vi "READ NEO values.vi"(8 "error in (no error)":errorcluster, 10 "RefName":string, 11 "MotorControlDevRef":T1) -> (0 "error out":errorcluster, 3 "MotorControlDevRef out":T1)   [LabVIEW 2020]
uses:
  <vilib>/Rock Robotics/WPI/MotorControl/WPI_MotorControlDeviceRef.ctl
  <vilib>/Rock Robotics/WPI/MotorControl/WPI_MotorControlType.ctl
  <vilib>/Rock Robotics/SystemInterfaces/DIO/FPGA_DIOPWMChannel.ctl
  <vilib>/Rock Robotics/WPI/PWM/WPI_PWMDeadband.ctl
  <vilib>/Rock Robotics/SystemInterfaces/DIO/FPGA_DIOChannel.ctl
  <vilib>/Rock Robotics/Network Tables/NT Write Number.vi
  <vilib>/Rock Robotics/Network Tables/NT Write Boolean.vi
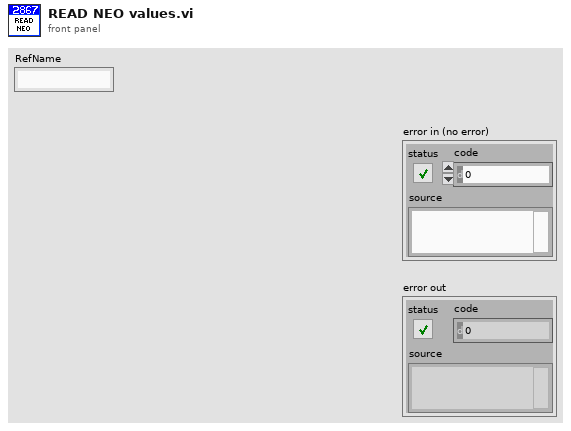
[diagram p1: front panel]
types:
  T1 = typedef "WPI_MotorControlDeviceRef.ctl" = cluster{"DeviceStatus":errorcluster, "Type":T2, "PWM":cluster{"PWM Channel":T3, "DeadBand":T4}, "CAN":cluster{"Device Number":u8, "SetOutput VI Ref":variant, "GetOutput VI Ref":variant, "Enable VI Ref":variant, "Disable VI Ref":variant, "Data":variant}, "Invert":bool, "DIO PWM":cluster{"PWM \"Enable\" Channel":T3, "DIOChannel":T5, "PWM Rate":dbl}}
  T2 = typedef "WPI_MotorControlType.ctl" = enum16{"PWM", "CAN", "DIO PWM"}
  T3 = typedef "FPGA_DIOPWMChannel.ctl" = enum8{"PWM 0", "PWM 1", "PWM 2", "PWM 3", "PWM 4", "PWM 5", "PWM 6", "PWM 7", "PWM 8", "PWM 9", "PWM MXP 0", "PWM MXP 1", "PWM MXP 2", "PWM MXP 3", "PWM MXP 4", "PWM MXP 5", "PWM MXP 6", "PWM MXP 7", "PWM MXP 8", "PWM MXP 9", "Invalid"}
  T4 = typedef "WPI_PWMDeadband.ctl" = cluster{"Name":string, "maxPositivePwm":i32, "minPositivePwm":i32, "centerPwm":i32, "maxNegativePwm":i32, "minNegativePwm":i32, "angularRange":u16}
  T5 = typedef "FPGA_DIOChannel.ctl" = enum8{"DIO 0", "DIO 1", "DIO 2", "DIO 3", "DIO 4", "DIO 5", "DIO 6", "DIO 7", "DIO 8", "DIO 9", "DIO MXP 0", "DIO MXP 1", "DIO MXP 2", "DIO MXP 3", "DIO MXP 4", "DIO MXP 5", "DIO MXP 6", "DIO MXP 7", "DIO MXP 8", "DIO MXP 9", "DIO MXP 10", "DIO MXP 11", "DIO MXP 12", "DIO MXP 13", "DIO MXP 14", "DIO MXP 15", "SPI Port CS1", "SPI Port CS2", "SPI Port CS3", "SPI Port MISO", "SPI Port MOSI", "Invalid"}
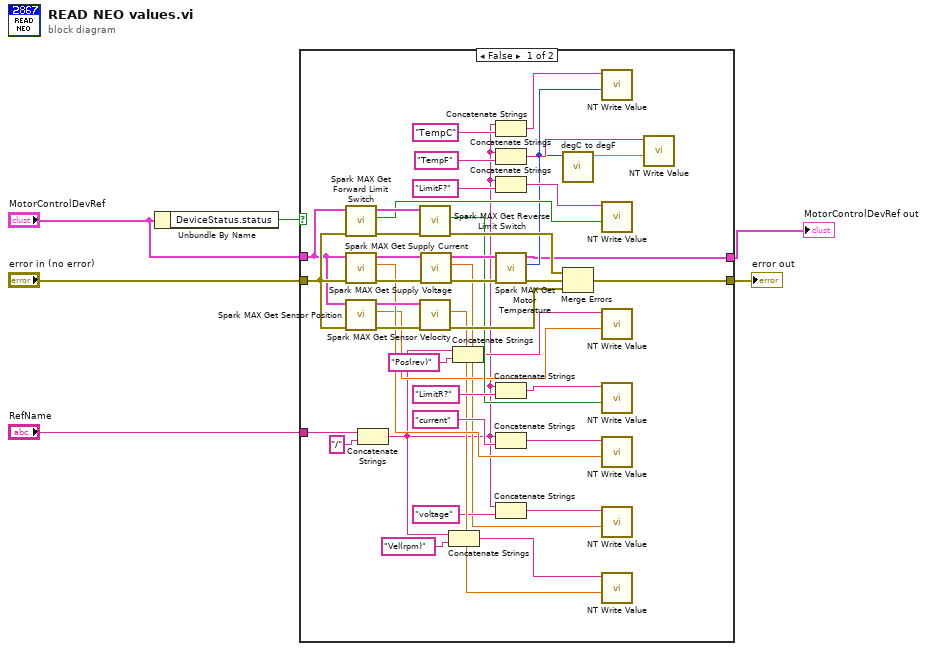
[diagram p0: block diagram]
diagram:
  n1 = Unbundle By Name("MotorControlDevRef") -> ("DeviceStatus.status"=w2:bool)
  n2 = case shown="False" w2 {
    tunnel: "RefName" -> [w48 _]
    tunnel: "error in (no error)" -> [w47 w49]
    tunnel: [w46 w49] -> w4
    tunnel: "MotorControlDevRef" -> [w45 w50]
    tunnel: [w7 w50] -> w1
    frame False {
      n3 = call <vilib>:"Spark MAX Get Forward Limit Switch.vi"("error in (no error)"=w47, "MotorControlDevRef in"=w45) -> ("error out"=w43:errorcluster, "Hard Limit Fwd"=w31:bool, "MotorControlDevRef out"=w40:T1)  [unwired: 6 in, 1 out]
      n4 = call <vilib>:"Spark MAX Get Supply Current.vi"("error in (no error)"=w47, "MotorControlDevRef in"=w45) -> ("error out"=w42:errorcluster, "Current"=w24:dbl, "MotorControlDevRef out"=w38:T1)  [unwired: 6 in, 1 out]
      n5 = call <vilib>:"Spark MAX Get Sensor Position.vi"("error in (no error)"=w47, "MotorControlDevRef in"=w45) -> ("error out"=w44:errorcluster, "Sensor Position"=w21:dbl, "MotorControlDevRef out"=w39:T1)  [unwired: 6 in, 1 out]
      n6 = Concatenate Strings(w48, "/" ("string")) -> (w8:string)
      n7 = call <vilib>:"Spark MAX Get Reverse Limit Switch.vi"("error in (no error)"=w43, "MotorControlDevRef in"=w40) -> ("error out"=w35:errorcluster, "Hard Limit Rev"=w27:bool)  [unwired: 6 in, 2 out]
      n8 = call <vilib>:"Spark MAX Get Sensor Velocity.vi"("error in (no error)"=w44, "MotorControlDevRef in"=w39) -> ("error out"=w36:errorcluster, "Sensor Velocity"=w18:dbl)  [unwired: 6 in, 2 out]
      n9 = call <vilib>:"Spark MAX Get Supply Voltage.vi"("error in (no error)"=w42, "MotorControlDevRef in"=w38) -> ("error out"=w41:errorcluster, "Voltage"=w15:dbl, "MotorControlDevRef out"=w37:T1)  [unwired: 6 in, 1 out]
      n10 = Concatenate Strings(w8, "Vel(rpm)" ("string")) -> (w20:string)
      n11 = Concatenate Strings(w8, "Pos(rev)" ("string")) -> (w23:string)
      n12 = Concatenate Strings(w8, "TempC" ("string")) -> (w14:string)
      n13 = Concatenate Strings(w8, "TempF" ("string")) -> (w12:string)
      n14 = Concatenate Strings(w8, "LimitF?" ("string")) -> (w32:string)
      n15 = call <vilib>:"Spark MAX Get Motor Temperature.vi"("error in (no error)"=w41, "MotorControlDevRef in"=w37) -> ("error out"=w34:errorcluster, "Motor Temperature"=w10:u8, "MotorControlDevRef out"=w7:T1)  [unwired: 6 in, 1 out]
      n16 = Concatenate Strings(w8, "LimitR?" ("string")) -> (w29:string)
      n17 = Concatenate Strings(w8, "current" ("string")) -> (w26:string)
      n18 = Concatenate Strings(w8, "voltage" ("string")) -> (w17:string)
      n19 = call "degC to degF.vi"("degreesC"=w10) -> ("degreesF"=w9:dbl)  [unwired: 10 in]
      n20 = Merge Errors(w35, w34, w36) -> (w46:errorcluster)
      n21 = call-poly <vilib>:"NT Write Value.vi"("Numeric"=w10, "Name"=w14) -> ()  [unwired: 9 in, 1 out]
      n22 = call-poly <vilib>:"NT Write Value.vi"("Boolean"=w31, "Name"=w32) -> ()  [unwired: 9 in, 1 out]
      n23 = call-poly <vilib>:"NT Write Value.vi"("Numeric"=w21, "Name"=w23) -> ()  [unwired: 9 in, 1 out]
      n24 = call-poly <vilib>:"NT Write Value.vi"("Boolean"=w27, "Name"=w29) -> ()  [unwired: 9 in, 1 out]
      n25 = call-poly <vilib>:"NT Write Value.vi"("Numeric"=w24, "Name"=w26) -> ()  [unwired: 9 in, 1 out]
      n26 = call-poly <vilib>:"NT Write Value.vi"("Numeric"=w15, "Name"=w17) -> ()  [unwired: 9 in, 1 out]
      n27 = call-poly <vilib>:"NT Write Value.vi"("Numeric"=w18, "Name"=w20) -> ()  [unwired: 9 in, 1 out]
      n28 = call-poly <vilib>:"NT Write Value.vi"("Numeric"=w9, "Name"=w12) -> ()  [unwired: 9 in, 1 out]
    }
    frame True {
    }
  }
  "error out" <- w4
  "MotorControlDevRef out" <- w1
